vi "_get_str.vi"(3 "错误输入（无错误）":errorcluster, 4 "写入缓冲区":string, 5 "VISA资源名称":refnum<visa-resource-name>) -> (0 "错误输出":errorcluster, 1 "读取缓冲区":string, 2 "VISA资源名称输出":refnum<visa-resource-name>)   [LabVIEW 2017]
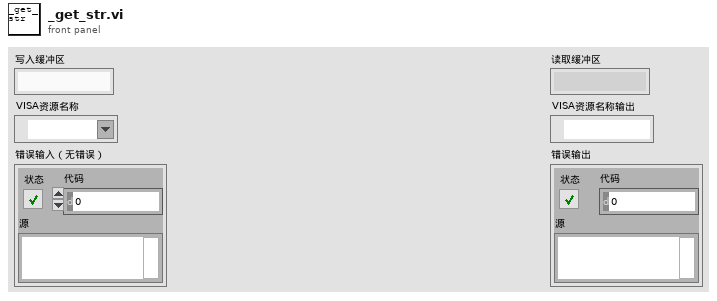
[diagram p1: front panel]
types:
  T1 = typedef "Semaphore RefNum" = refnum<k1>
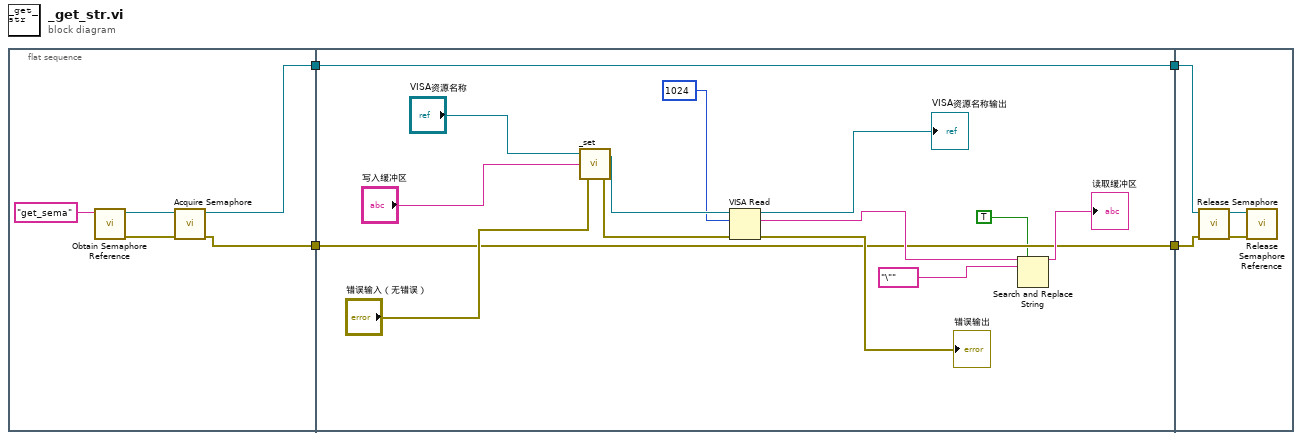
[diagram p0: block diagram]
diagram:
  n1 = flat-sequence {
    tunnel: [w7] -> w3
    tunnel: [w6] -> w2
    tunnel: [w12] -> w4
    tunnel: w3 -> [w12]
    tunnel: w2 -> [w11]
    tunnel: [w11] -> w1
    tunnel: w4 -> [w25]
    tunnel: w1 -> [w24]
    frame #0 {
      n2 = call <vilib>:"Obtain Semaphore Reference.vi"("name (unnamed)"="get_sema") -> ("error out"=w8:errorcluster, "semaphore"=w9:T1)  [unwired: 4 in, 1 out]
      n3 = call <vilib>:"Acquire Semaphore.vi"("error in (no error)"=w8, "semaphore"=w9) -> ("error out"=w7:errorcluster, "semaphore out"=w6:T1)  [unwired: 3 in, 1 out]
    }
    frame #1 {
      n4 = call "_set.vi"("错误输入（无错误）"="错误输入（无错误）", "写入缓冲区"="写入缓冲区", "VISA资源名称输出 2"="VISA资源名称") -> ("错误输出"=w19:errorcluster, "VISA资源名称输出"=w20:refnum<visa-resource-name>)
      n5 = VISA Read(VISA resource name=w20, byte count=u32 1024 ("字节总数"), error in (no error)=w19) -> (VISA resource name out=→"VISA资源名称输出":refnum<visa-resource-name>, read buffer=w15:string, error out=→"错误输出":errorcluster)  [unwired: 1 out]
      n6 = Search and Replace String(replace all?=TRUE ("替换全部？(F)"), input string=w15, search string="\"" ("搜索字符串")) -> (result string=→"读取缓冲区":string)  [unwired: 5 in, 3 out]
    }
    frame #2 {
      n7 = call <vilib>:"Release Semaphore.vi"("error in (no error)"=w25, "semaphore"=w24) -> ("error out"=w27:errorcluster, "semaphore out"=w26:T1)  [unwired: 4 in]
      n8 = call <vilib>:"Release Semaphore Reference.vi"("error in (no error)"=w27, "semaphore"=w26) -> ()  [unwired: 8 in, 2 out]
    }
  }
